vi "Start End time VI.vi"(11 "Boolean frame energy":i16[](array[numeric])) -> (0 "Smooth Energy":dbl[](graph), 1 "End Time":dbl, 2 "Length":dbl, 3 "Start Time":dbl, 5 "max index":dbl, 7 "min index":dbl)   [LabVIEW 2013]
uses:
  <vilib>/Analysis/NI_AALBase.lvlib
  <vilib>/Analysis/NI_AAL_SigProc.lvlib
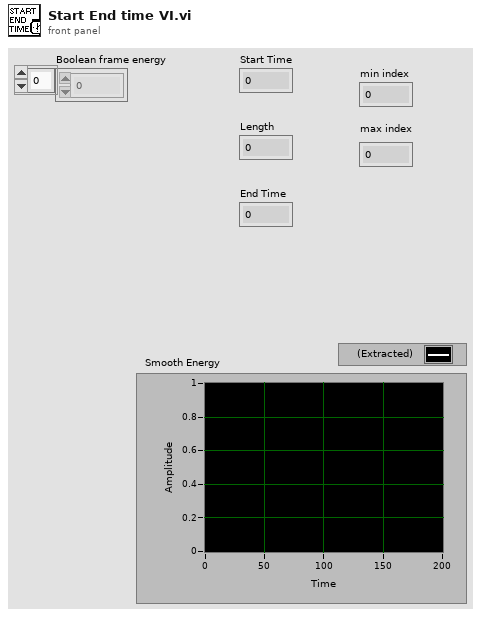
[diagram p1: front panel]
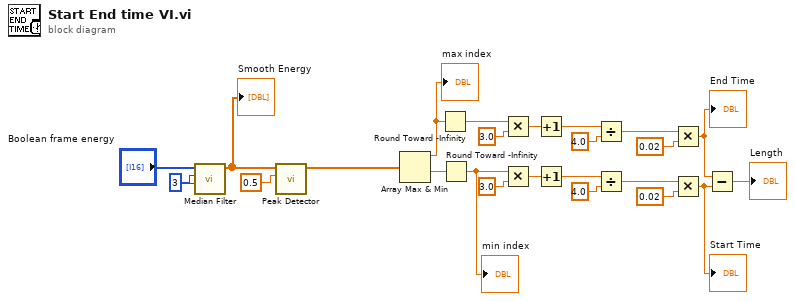
[diagram p0: block diagram]
diagram:
  w6 = 3 ("right rank")
  n1 = call <vilib>:"Median Filter.vi"("right rank"=w6, "left rank"=w6, "X"="Boolean frame energy") -> ("Filtered X"=w3:dbl[])  [unwired: 7 in, 1 out]
  "Smooth Energy" <- w3
  n2 = call <vilib>:"Peak Detector.vi"("threshold"=0.5, "X"=w3) -> ("Locations"=w5:dbl[])  [unwired: 5 in, 4 out]
  n3 = Array Max & Min(array=w5) -> (max value=w7:dbl, min value=w2:dbl)  [unwired: 2 out]
  "max index" <- w7
  n4 = Round Toward -Infinity(1:w7) -> (0:w21:dbl)
  n5 = Round Toward -Infinity(1:w2) -> (0:w1:dbl)
  "min index" <- w1
  n6 = Multiply(x=w21, y=3.0) -> (x*y=w10:dbl)
  n7 = Multiply(x=w1, y=3.0) -> (x*y=w19:dbl)
  n8 = Increment(x=w10) -> (x+1=w11:dbl)
  n9 = Increment(x=w19) -> (x+1=w18:dbl)
  n10 = Divide(x=w11, y=4.0) -> (x/y=w13:dbl)
  n11 = Divide(x=w18, y=4.0) -> (x/y=w16:dbl)
  n12 = Multiply(x=w13, y=0.02) -> (x*y=w22:dbl)
  "End Time" <- w22
  n13 = Multiply(x=w16, y=0.02) -> (x*y=w23:dbl)
  "Start Time" <- w23
  n14 = Subtract(x=w22, y=w23) -> (x-y=→"Length":dbl)
